vi "Delete Menu.vi"(5 "Submenu Tags Validated":string[](array[string]), 7 "Submenu Tags to Check":string[](array[string]), 8 "error in (no error)":errorcluster, 11 "MenuRef":refnum<k9>) -> (0 "error out":errorcluster, 3 "Dup MenuRef":refnum<k9>)   [LabVIEW 2017, in "3D Plot.lvclass"]
uses:
  <vilib>/Math Plots/3D Math Plots/3D Plot/3D Plot/3D Plot.lvclass
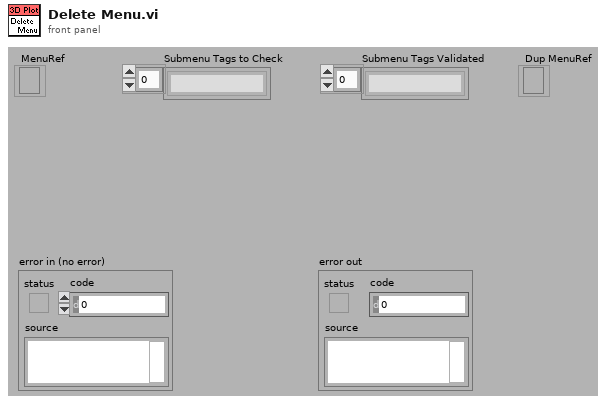
[diagram p1: front panel]
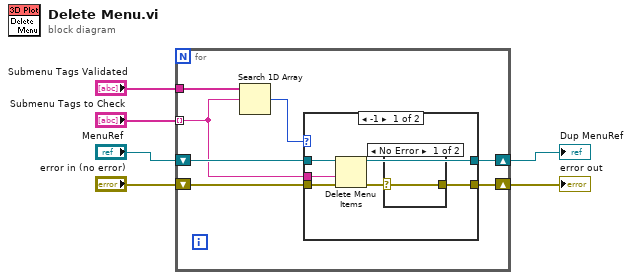
[diagram p0: block diagram]
diagram:
  n1 = for {
    tunnel: "Submenu Tags Validated" -> [w11]
    shift-right: [w12] -> w5
    shift-left: "MenuRef" -> [w13]
    tunnel: "Submenu Tags to Check" -> [w9] mode=indexing
    shift-right: [w7] -> w6
    shift-left: "error in (no error)" -> [w8]
    n2 = Search 1D Array(1D array=w11, element=w9) -> (index of element=w10:i32)  [unwired: 1 out]
    n3 = case shown="-1" w10 {
      tunnel: w13 -> [w19 w22]
      tunnel: [w18 w22] -> w12
      tunnel: w9 -> [w16 _]
      tunnel: w8 -> [w17 w21]
      tunnel: [w14 w21] -> w7
      frame -1 {
        n4 = Delete Menu Items(6:w17, 7:w16, 9:w19) -> (0:w15:errorcluster, 3:w18:refnum<k9>)  [unwired: 1 out]
        n5 = case shown="No Error" w15 {
          selector: w15 -> [w20 _]
          tunnel: [w20 _] -> w14
          frame No Error {
          }
          frame Error {
          }
        }
      }
      frame Default {
      }
    }
  }
  "error out" <- w6
  "Dup MenuRef" <- w5
